vi "String to positions.vi"(11 "string":string) -> (3 "Array":dbl[](array[numeric]))   [LabVIEW 2020, in "Arduino-Adafruit stepper.lvlib"]
uses:
  Arduino-Adafruit stepper.lvlib
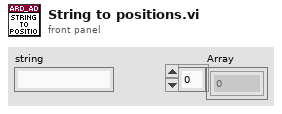
[diagram p1: front panel]
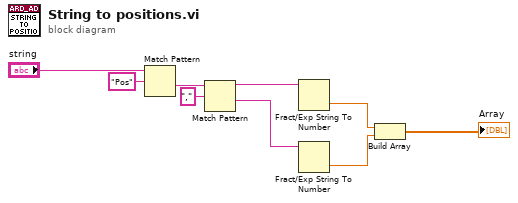
[diagram p0: block diagram]
diagram:
  n1 = Match Pattern(string="string", regular expression="Pos") -> (after substring=w3:string)  [unwired: 1 in, 3 out]
  n2 = Match Pattern(string=w3, regular expression=",") -> (before substring=w6:string, after substring=w1:string)  [unwired: 1 in, 2 out]
  n3 = Fract/Exp String To Number(string=w6) -> (number=w7:dbl)  [unwired: 3 in, 1 out]
  n4 = Fract/Exp String To Number(string=w1) -> (number=w8:dbl)  [unwired: 3 in, 1 out]
  n5 = Build Array(w7, w8) -> (→"Array":dbl[])
